vi "Trigger Generator Demo.vi"() -> ()   [LabVIEW 2015]
doc: "I. Description:\nThis example demonstrates how to generate a finite retriggerable digital pulse train from a Counter to be used as the clock for Analog Input. This example utilizes two counters.\n\nII. Instructions for Running:\n1. Select the physical channel to correspond to where your signal is input on the DAQ device.\n2. Enter the minimum and maximum signal ranges.\nNote: For better accuracy, try to match the input range to the expected voltage level of the measured signal.\n3. Select the Counter Channel which corresponds to the counter you want to generate your AI clock from.\n4. Select the Source of the Clock for the acquisition as the output of the counter you chose in step 3.\n5. Set the Rate at which the counter will generate.\nNote: The Rate should be at least twice as fast as the maximum frequency component of the signal being acquired.\n6. Enter the number of Samples per Channel to acquire. This will also be the number of pulses generated by the counter.\n7. Select the Source of the Digital Start Trigger for the acquisition.\n8. Select the edge, rising or falling, on which to trigger.\n\nIII. Block Diagram Steps:\n1. Create an analog input voltage channel. Also, create a Counter Output channel to produce a Pulse in terms of Frequency. If the Idle State of the pulse is set to low the first transition of the generated signal is from low to high.\n2. Define the parameters for an External Clock Source. Additionally, define the sample mode to be continuous. Also, use the DAQmx Timing VI (Implicit) to configure the duration of the pulse generation and the number of pulses to generate.\n3. Use the DAQmx Trigger VI to configure a counter trigger to start on a digital edge.\n4. Configure a buffer which is 1000 plus the number of samples per channel. This is necessary when simulating retriggerable finite transfers with a continuous acquisition because DMA needs a slightly larger buffer than the Samples per Channel. \n5. Use a DAQmx Trigger Property Node to set the operation for retriggerable.\n6. Call the Start VI to begin the acquisition and to arm the counter which begins the pulse train generation.\n7. Use the DAQ Read property node --> AvailSampPerChan to see how many samples have been acquired. If 'Samples per Channel' number of samples have been acquired, as you can set on the front panel, then Read the data, otherwise continue looping. This allows the user to stop the program by pressing the 'STOP' button at any time. \n8. Read the waveform data in a loop until the user hits the stop button or an error occurs.\nNote: This example reads data from one or more channels and returns an array of data. Use the Index Array function to access an individual channel of data.\n9. Call the Clear Task VI to clear the counter Task.\n10. Call the Clear Task VI to clear the AI Task.\n11. Use the popup dialog box to display an error if any.\n\nIV. I/O Connections Overview:\nMake sure your signal input terminal matches the Physical Channel I/O control. Note that there is no external wiring necessary to connect the counter output to the AI clock input. For further connection information, refer to your hardware reference manual."
uses:
  <vilib>/DAQmx/create/channels.llb/DAQmx Create Channel (DI-Digital Input).vi
  <vilib>/DAQmx/configure/timing.llb/DAQmx Timing (Change Detection).vi
  <vilib>/DAQmx/create/channels.llb/DAQmx Create Channel (CO-Pulse Generation-Ticks).vi
  <vilib>/DAQmx/configure/trigger.llb/DAQmx Start Trigger (Digital Edge).vi
  <resource>/objmgr/daqmx.rc
panel:
  in  "Edge source":tag="PXI1Slot2/port0/line0"
  in  "Start source":tag="/PXI1Slot2/ChangeDetectionEvent"
  in  "TTL duration (us)":dbl=100.0
  in  "Stop":bool caption="stop"
  in  "Counter":tag="PXI1Slot2/ctr0"
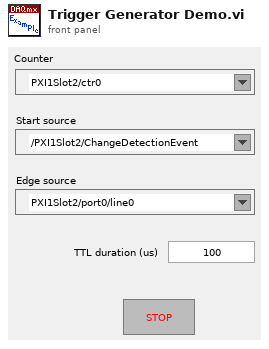
[diagram p1: front panel]
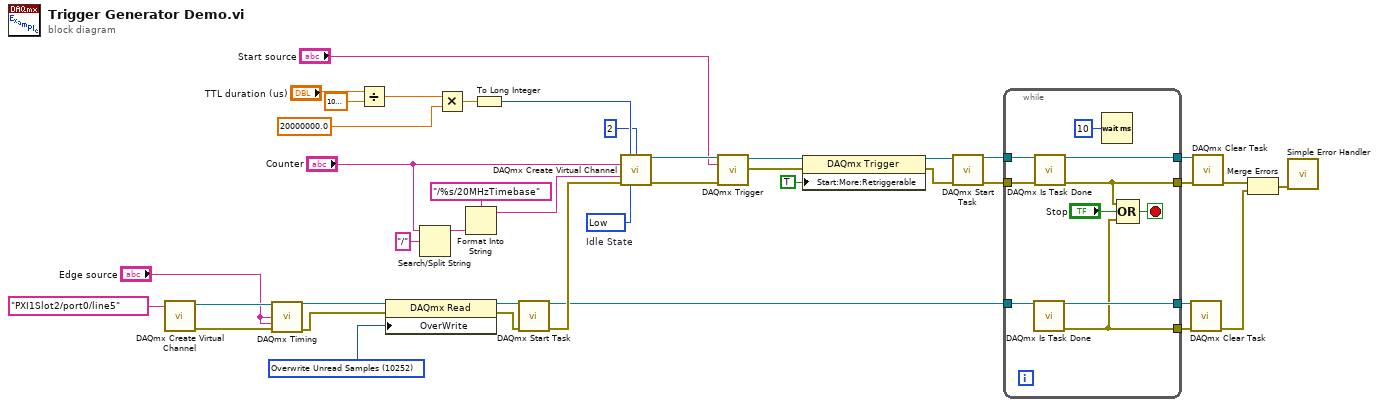
[diagram p0: block diagram]
diagram:
  w12 = 10252 items=["Overwrite Unread Samples"=10252, "Do Not Overwrite Unread Samples"=10159] ("OverWrite")
  w41 = 10214 items=["High"=10192, "Low"=10214]  # Idle State
  n1 = call-poly <vilib>:"DAQmx Create Virtual Channel.vi"("lines"=tag "PXI1Slot2/port0/line5") -> ("task out"=w14:refnum<k21>, "error out"=w13:errorcluster)  [unwired: 13 in]
  n2 = call-poly <vilib>:"DAQmx Timing.vi"("task/channels in"=w14, "rising edge physical channels"="Edge source", "falling edge physical channels"="Edge source", "error in"=w13) -> ("task out"=w11:refnum<k21>, "error out"=w10:errorcluster)  [unwired: 10 in]
  n3 = Divide(x="TTL duration (us)", y=1000000.0) -> (x/y=w25:dbl)
  n4 = property class="DAQmx Read"(reference=w11, error in=w10, "OverWrite"=w12) -> (reference out=w9:refnum<k21>, error out=w8:errorcluster)
  n5 = Search/Split String(string="Counter", search string/char (-)="/") -> (substring before match=w30:string)  [unwired: 1 in, 2 out]
  n6 = Multiply(x=w25, y=20000000.0) -> (x*y=w23:dbl)
  n7 = Format Into String(format string="/%s/20MHzTimebase", w30) -> (resulting string=w28:string)  [unwired: 2 in, 1 out]
  n8 = To Long Integer(number=w23) -> (32bit integer=w21:i32)
  n9 = call <vilib>:"DAQmx Start Task.vi"("task/channels in"=w9, "error in"=w8) -> ("task out"=w5:refnum<k21>, "error out"=w7:errorcluster)  [unwired: 12 in]
  n10 = call-poly <vilib>:"DAQmx Create Virtual Channel.vi"("high ticks"=w21, "low ticks"=u32 2, "counter"="Counter", "source of ticks"=w28, "error in"=w7, "idle state"=w41) -> ("task out"=w18:refnum<k21>, "error out"=w17:errorcluster)  [unwired: 8 in]
  n11 = call-poly <vilib>:"DAQmx Trigger.vi"("task/channels in"=w18, "source"="Start source", "error in"=w17) -> ("task out"=w40:refnum<k21>, "error out"=w39:errorcluster)  [unwired: 11 in]
  n12 = property class="DAQmx Trigger"(reference=w40, error in=w39, "Start:More:Retriggerable"=TRUE) -> (reference out=w38:refnum<k21>, error out=w37:errorcluster)
  n13 = call <vilib>:"DAQmx Start Task.vi"("task/channels in"=w38, "error in"=w37) -> ("task out"=w36:refnum<k21>, "error out"=w32:errorcluster)  [unwired: 12 in]
  n14 = while {
    tunnel: [w48] -> w35
    tunnel: w36 -> [w49]
    tunnel: [w47] -> w34
    tunnel: w32 -> [w46]
    tunnel: w5 -> [w44]
    tunnel: [w43] -> w4
    tunnel: [w42] -> w3
    stop <- w50 stop-if-true
    n15 = call <vilib>:"DAQmx Is Task Done.vi"("task/channels in"=w44) -> ("task out"=w43:refnum<k21>, "error out"=w42:errorcluster)  [unwired: 12 in, 1 out]
    n16 = call <vilib>:"DAQmx Is Task Done.vi"("task/channels in"=w49, "error in"=w46) -> ("task out"=w48:refnum<k21>, "error out"=w47:errorcluster)  [unwired: 11 in, 1 out]
    n17 = Wait (ms)(milliseconds to wait=u32 10) -> ()  [unwired: 1 out]
    n18 = Compound Arithmetic op=OR(w47, "Stop", w42) -> (w50:bool)
  }
  n19 = call <vilib>:"DAQmx Clear Task.vi"("task in"=w4, "error in"=w3) -> ("error out"=w1:errorcluster)  [unwired: 13 in]
  n20 = call <vilib>:"DAQmx Clear Task.vi"("task in"=w35, "error in"=w34) -> ("error out"=w33:errorcluster)  [unwired: 13 in]
  n21 = Merge Errors(w33, w1) -> (w2:errorcluster)
  n22 = call <vilib>:"Simple Error Handler.vi"("error in (no error)"=w2) -> ()  [unwired: 4 in, 5 out]
